vi "EnumerateStepTypes.vi"(8 "error in (no error)":errorcluster, 11 "Step Classes Folder":path) -> (0 "error out":errorcluster, 3 "Step Names":string[](array[string]))   [LabVIEW 2015, in "CleanupCategoryNode.lvclass"]
uses:
  CleanupCategoryNode.lvclass
  <vilib>/NI/Configuration Framework/class discovery singleton/class discovery singleton.lvlib
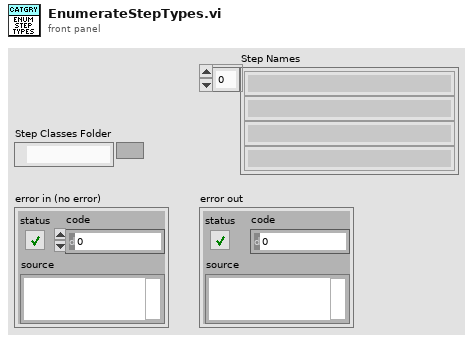
[diagram p1: front panel]
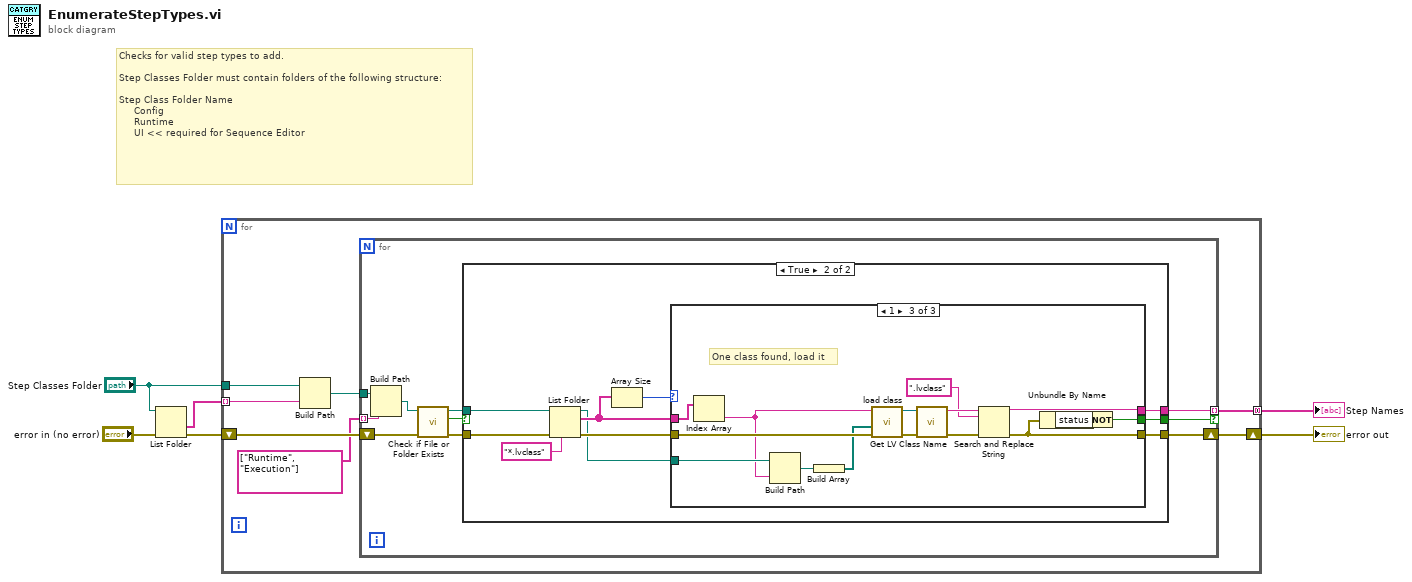
[diagram p0: block diagram]
diagram:
  # "Checks for valid step types to add.\n\nStep Classes Folder must contain folders of the following structure:\n\nStep Class Folder Name\n     Config\n     Runtime\n     UI << required for Sequence Editor"
  n1 = List Folder(path="Step Classes Folder", error in="error in (no error)") -> (folder names=w3:string[], error out=w6:errorcluster)  [unwired: 2 in, 2 out]
  n2 = for {
    shift-right: [w9] -> w4
    shift-left: w6 -> [w13]
    tunnel: w3 -> [w11] mode=indexing
    tunnel: "Step Classes Folder" -> [w12]
    tunnel: [w8] -> w1 mode=concatenating
    n3 = Build Path(base path=w12, name or relative path=w11) -> (appended path=w10:path)
    n4 = for {
      tunnel: w10 -> [w22]
      tunnel: [w16] -> w8 mode=indexing if=w14
      tunnel: string[] ["Runtime", "Execution"] ("name or relative path") -> [w15] mode=indexing
      shift-right: [w18] -> w9
      shift-left: w13 -> [w23]
      n5 = Build Path(base path=w22, name or relative path=w15) -> (appended path=w21:path)
      n6 = call <vilib>:"Check if File or Folder Exists.vi"("error in (no error)"=w23, "path"=w21) -> ("error out"=w17:errorcluster, "file or folder exists?"=w20:bool, "dup path"=w19:path)  [unwired: 7 in]
      n7 = case shown="True" w20 {
        tunnel: w19 -> [_ w33]
        tunnel: [w24 w30] -> w18
        tunnel: w17 -> [w24 w34]
        tunnel: [_ w26] -> w16
        tunnel: [_ w25] -> w14
        frame False {
          # "No UI folder found for current step folder"
        }
        frame True {
          n8 = List Folder(path=w33, pattern="*.lvclass", error in=w34) -> (path out=w27:path, filenames=w29:string[], error out=w31:errorcluster)  [unwired: 1 in, 1 out]
          n9 = Array Size(array=w29) -> (size(s)=w28:i32)
          n10 = case shown="1" w28 {
            tunnel: w31 -> [w35 w36 w51]
            tunnel: [w35 w36 w40] -> w30
            tunnel: w29 -> [_ _ w49]
            tunnel: w27 -> [_ _ w48]
            tunnel: [_ _ w38] -> w26
            tunnel: [_ _ w42] -> w25
            frame 0 {
              # "No classes found in folder, skip"
            }
            frame Default {
              # "More than 1 class found in folder.\nThere should not be more than \none class per UI folder, throw error?"
            }
            frame 1 {
              # "One class found, load it"
              n11 = Index Array(array=w49) -> (element=w47:string)  [unwired: 1 in]
              n12 = Build Path(base path=w48, name or relative path=w47) -> (appended path=w46:path)
              n13 = Build Array(w46) -> (w45:path[])
              n14 = call <vilib>:"load class.vi"("error in"=w51, "available class paths"=w45, "Class Name"=w47) -> ("error out"=w50:errorcluster, "Object Out"=w44:refnum<class>)  [unwired: 7 in]
              n15 = call <vilib>:"Get LV Class Name.vi"("error in (no error)"=w50, "object"=w44) -> ("error out"=w41:errorcluster, "class name"=w39:string)  [unwired: 8 in]
              n16 = Search and Replace String(input string=w39, search string=".lvclass", error in=w41) -> (result string=w38:string, error out=w40:errorcluster)  [unwired: 5 in, 2 out]
              n17 = Unbundle By Name(w40) -> ("status"=w43:bool)
              n18 = Not(x=w43) -> (.not. x?=w42:bool)
            }
          }
        }
      }
    }
  }
  "Step Names" <- w1
  "error out" <- w4
